vi "FilePaths.vi"(8 "error in":errorcluster) -> (0 "error out":errorcluster, 2 "paths":T1)   [LabVIEW 2013, in "vi mod UI.lvlib"]
uses:
  vi mod UI.lvlib
  Controls/FilePaths.ctl
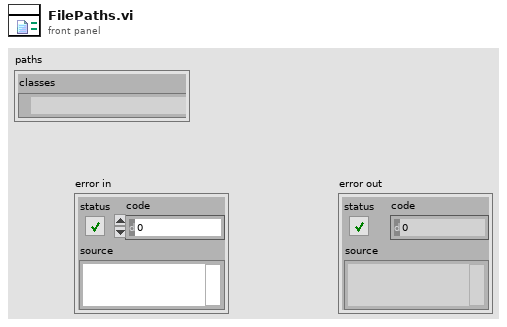
[diagram p1: front panel]
types:
  T1 = typedef "vi mod UI.lvlib/FilePaths.ctl" = cluster{"classes":path}
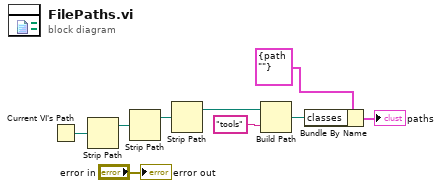
[diagram p0: block diagram]
diagram:
  n1 = Current VI's Path() -> (path=w6:path)
  n2 = Strip Path(path=w6) -> (stripped path=w4:path)  [unwired: 1 out]
  n3 = Strip Path(path=w4) -> (stripped path=w5:path)  [unwired: 1 out]
  n4 = Strip Path(path=w5) -> (stripped path=w3:path)  [unwired: 1 out]
  n5 = Build Path(base path=w3, name or relative path="tools") -> (appended path=w1:path)
  n6 = Bundle By Name(cluster=T1 {"classes"=path ""} ("Cluster 2"), "classes"=w1) -> (→"paths":T1)
  "error out" <- "error in"
